vi "optelling_afslagen_deel2(SubVI).vi"(10 "Numeric":i32, 11 "OK Button":bool) -> (2 "Numeric 2":i32)   [LabVIEW 2019]
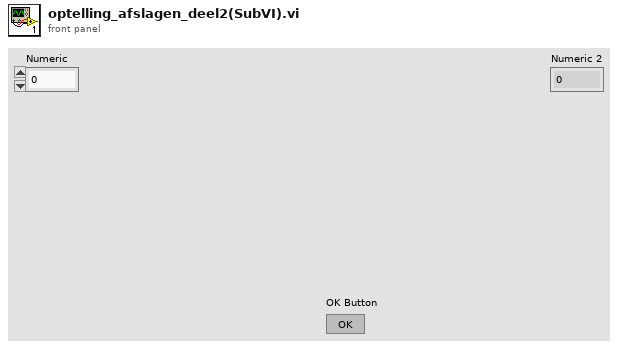
[diagram p1: front panel]
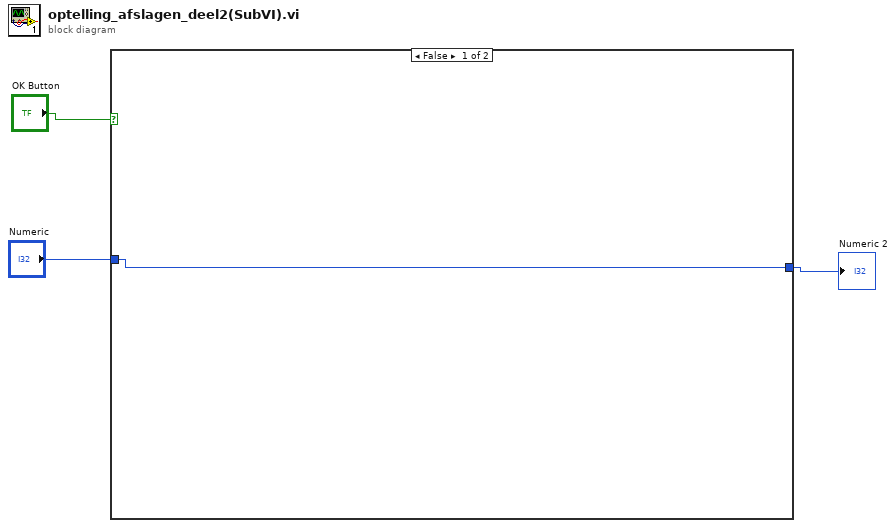
[diagram p0: block diagram]
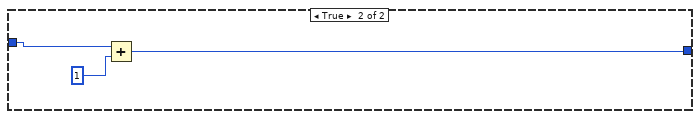
[diagram p2: hidden frame]
diagram:
  n1 = case shown="False" "OK Button" {
    tunnel: "Numeric" -> [w4 w6]
    tunnel: [w4 w5] -> w1
    frame False {
    }
    frame True {
      n2 = Add(x=w6, y=1) -> (x+y=w5:i32)
    }
  }
  "Numeric 2" <- w1
